vi "test_LoadFrameEditorFile_v2.vi"(11 "BIN file path":path=path "C:/Users/Administrator/Desktop/git/niveristand-aim-arinc664-custom-device/Docs/User Guide/Assets/standard_frames_udp.bin") -> (0 "error out":errorcluster)   [LabVIEW 2020]
uses:
  <instrlib>/AIM GmbH/_AIM 664/helpers/EthFrameManagement/EthFrameManagement.lvlib
  Frame Configuration/controls/Type of Payload.ctl
  Frame Configuration/controls/Payload Record Type.ctl
  Import/AIM ARINC 664 Import.lvlib
  <instrlib>/AIM GmbH/_AIM 664/helpers/EthFrameManagement/controls/ehternetFrame_type.ctl
  <instrlib>/AIM GmbH/_AIM 664/helpers/EthFrameManagement/controls/IPFrame_type.ctl
  <instrlib>/AIM GmbH/_AIM 664/helpers/EthFrameManagement/controls/UDPFrame_type.ctl
  Shared/frame_tx_generic_seqNumberInit.ctl
  Shared/frame_tx_generic_seqNumberOffset.ctl
  Shared/frame_tx_generic.ctl
  <vilib>/NI/NI VeriStand Encoding and Decoding/Encoding.ctl
  <vilib>/NI/NI VeriStand Encoding and Decoding/Encoding and Decoding.lvlib
  Shared/frame_parameter_definition.ctl
  Shared/frame_parameter.ctl
panel:
  out "Frame Headers":T1[](array[typedef]) {"Frame header"."SequenceNumberOffset" items=["FDX_TX_FRAME_SEQ_OFFS_AUTO"=65535]; "Frame header"."SequenceNumberInit" items=["FDX_TX_FRAME_SEQ_INIT_AUTO"=65535, "FDX_TX_FRAME_SEQ_OFF"=65533]; "Frame header"."PhysErrorInjection" items=["FDX_TX_FRAME_ERR_OFF", "FDX_TX_FRAME_ERR_CRC", "FDX_TX_FRAME_ERR_ALI", "FDX_TX_FRAME_ERR_PRE", "FDX_TX_FRAME_ERR_PHY"]; "Frame header"."PayloadGenerationMode" items=["FDX_TX_FRAME_PGM_USER", "FDX_TX_FRAME_PGM_IP_PART", "FDX_TX_FRAME_PGM_IP_PART_TT", "FDX_TX_FRAME_PGM_IP_FULL", "FDX_TX_FRAME_PGM_IP_FULL_TT"]; "Frame header"."PayloadBufferMode" items=["FDX_TX_FRAME_PBM_STD", "FDX_TX_FRAME_PBM_MAC", "FDX_TX_FRAME_PBM_UDP", "FDX_TX_FRAME_PBM_FULL"]; "Frame header"."NetSelect" items=["FDX_TX_FRAME_DLY_A"=0, "FDX_TX_FRAME_DLY_B"=1, "FDX_TX_FRAME_BOTH "=3, "FDX_TX_FRAME_ONLY_A"=4, "FDX_TX_FRAME_ONLY_B "=5]; "Frame header"."FrameStartMode" items=["FDX_TX_FRAME_START_IFG", "FDX_TX_FRAME_START_PGWT", "FDX_TX_FRAME_START_TRG", "FDX_TX_FRAME_START_TRG_D"]}
  in  "port index":i32
  in  "frame index":i32
  in  "XML file path":path=path "C:/Users/Administrator/Desktop/git/niveristand-aim-arinc664-custom-device/Docs/User Guide/Assets/Loopback_TxGen_RxMonitor.xml"
  out "data":cluster{"FrameID":string, "frame_record":T7}[](array[cluster])=[{"FrameID"="Payload1", "frame_record"={"Data"=[3, 0, 0, 0, 0, 60, 2, 0, 0, 1, 33, 32, 8, 0, 69, 0, 0, 45, 0, 0, 64, 0, 1, 17, 109, 162, 10, 1, 33, 1, 224, 224, 0, 60, 0, 1, 0, 1, 0, 25, 0, 0, 0, 0, 0, 0, 0, 0, 0, 0, 0, 0, 0, 0, 0, 0, 0, 0, 0, 0, 0, 0, 0, 0], "Type of Frame"=1}}, {"FrameID"="Payload2", "frame_record"={"Data"=[3, 0, 0, 0, 0, 60, 2, 0, 0, 1, 33, 32, 8, 0, 69, 0, 0, 45, 0, 0, 64, 0, 1, 17, 109, 162, 10, 1, 33, 1, 224, 224, 0, 60, 0, 1, 0, 1, 0, 25, 0, 0, 65, 66, 67, 68, 69, 70, 71, 72, 73, 74, 75, 76, 77, 78, 79, 80, 81, 0, 0, 0, 0, 0], "Type of Frame"=1}}, {"FrameID"="Payload3", "frame_record"={"Data"=[10, 10, 10, 10, 10, 10, 10, 10, 10, 10, 10, 10, 10, 10, 10, 10, 10], "Type of Frame"=2}}] {"frame_record"."Type of Frame" items=["Raw Frame", "UDP/IP Tx Gen", "Tx UDP"]; "frame_record"."Data" format="%.0x"}
  out "dst ip":string="224.224.0.60"
  out "src ip":string="10.1.33.1"
  out "size(s)":i32=22
  out "UDP header":T9={"Source Port"=1, "Dest Port"=1, "Lenght"=25, "Checksum"=0}
  out "IP header":T10={"Version"=4, "IHL"=5, "ToS"=0, "Length"=45, "ID"=0, "CtlFlags"=2, "FragOffset"=0, "TTL"=1, "Protocol"=17, "Checksum"=28066, "Source IP"=167846145, "Dest IP"=3772776508} {"CtlFlags" format="%.0b"; "Dest IP" format="%.0x"; "Source IP" format="%.0x"; "Checksum" format="%.0x"; "TTL" format="%.0x"; "FragOffset" format="%.0x"; "ID" format="%.0x"; "Length" format="%.0x"; "ToS" format="%.0x"; "IHL" format="%.0x"; "Version" format="%.0x"}
  out "UDP Header Only":u8[](array[numeric])=[0, 1, 0, 1, 0, 25, 0, 0]
  out "IP Header Only":u8[](array[numeric])=[69, 0, 0, 45, 0, 0, 64, 0, 1, 17, 109, 162, 10, 1, 33, 1, 224, 224, 0, 60] format="%.0x"
  out "Ethernet header":T11={"Dest MAC"=[3, 0, 0, 0, 0, 60], "Src MAC"=[2, 0, 0, 1, 33, 32], "EtherType"=2048} {"EtherType" format="%04x"; "Src MAC" format="%02x"; "Dest MAC" format="%.0b"}
  out "MAC Header Only":u8[](array[numeric])=[3, 0, 0, 0, 0, 60, 2, 0, 0, 1, 33, 32, 8, 0] format="%.0x"
  out "payload":u8[](array[numeric]) format="%.0x"
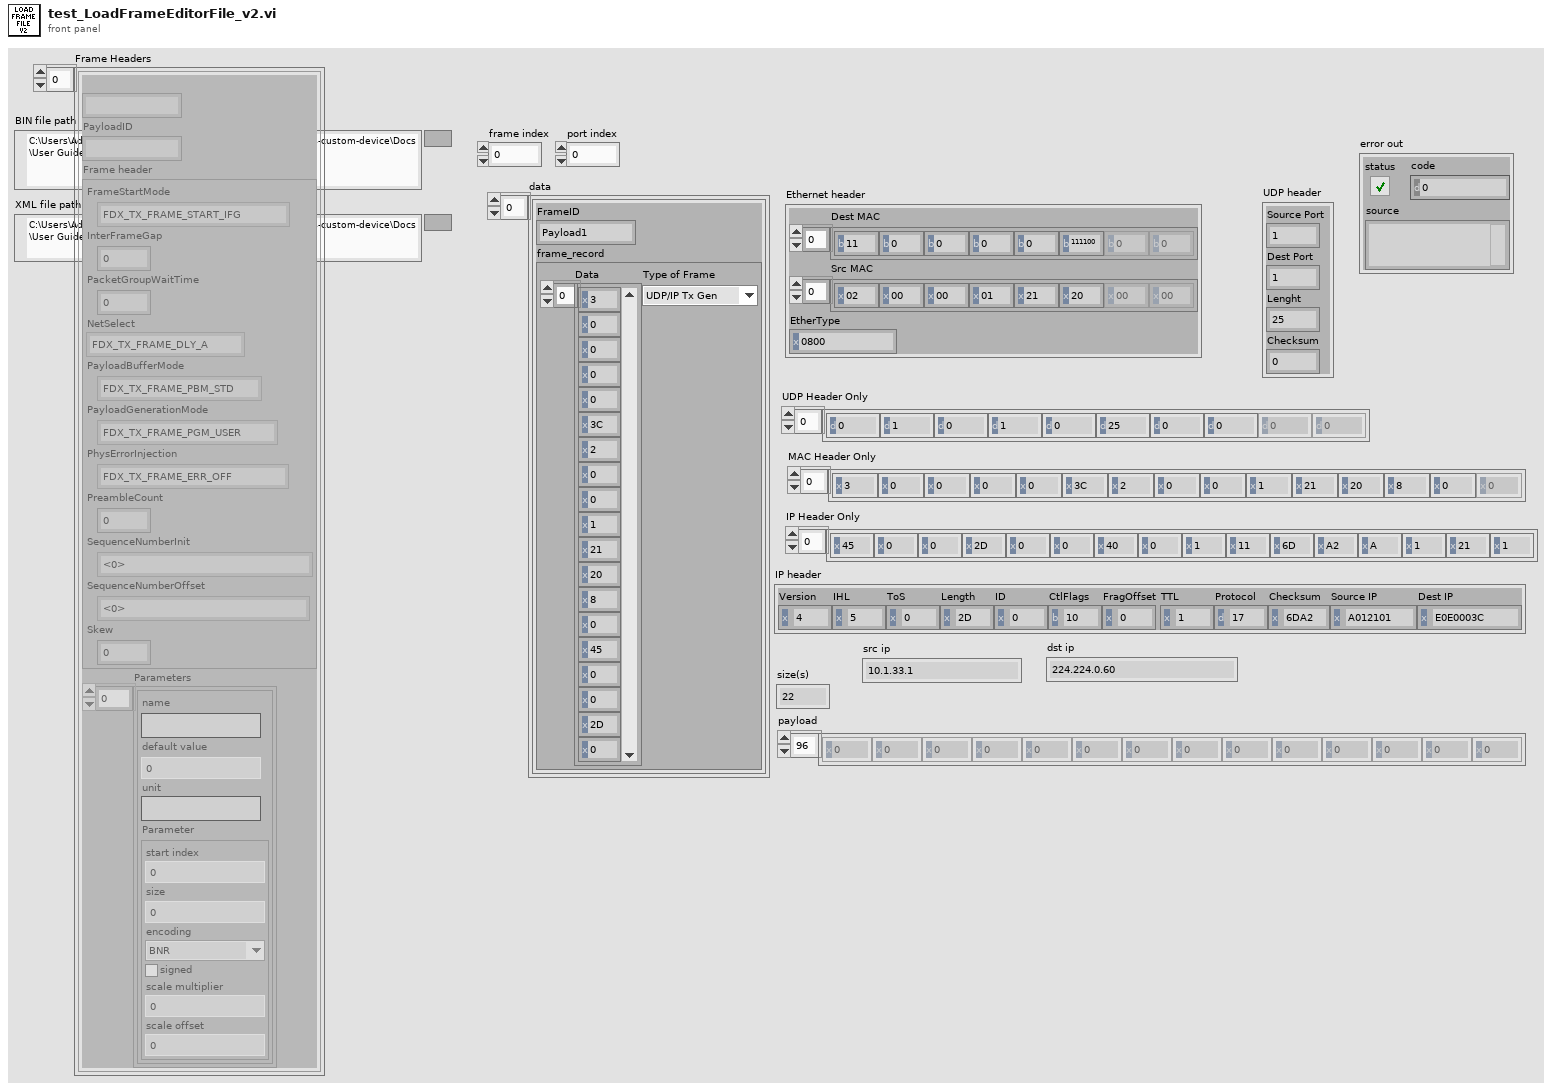
[diagram p1: front panel]
types:
  T1 = typedef "AIM ARINC 664 Import.lvlib/frame_tx_generic.ctl" = cluster{"FrameID":string, "PayloadID":string, "Frame header":cluster{"FrameStartMode":i32, "InterFrameGap":i32, "PacketGroupWaitTime":i32, "NetSelect":u32, "PayloadBufferMode":i32, "PayloadGenerationMode":i32, "PhysErrorInjection":i32, "PreambleCount":i32, "SequenceNumberInit":T2, "SequenceNumberOffset":T3, "Skew":i32}, "Parameters":T4[]}
  T2 = typedef "AIM ARINC 664 Import.lvlib/frame_tx_generic_seqNumberInit.ctl" = i32
  T3 = typedef "AIM ARINC 664 Import.lvlib/frame_tx_generic_seqNumberOffset.ctl" = i32
  T4 = typedef "AIM ARINC 664 Import.lvlib/frame_parameter.ctl" = cluster{"name":string, "default value":dbl, "unit":string, "Parameter":T5}
  T5 = typedef "AIM ARINC 664 Import.lvlib/frame_parameter_definition.ctl" = cluster{"start index":i32, "size":i32, "encoding":T6, "signed":bool, "scale multiplier":dbl, "scale offset":dbl}
  T6 = typedef "Encoding and Decoding.lvlib/Encoding.ctl" = enum16{"BNR", "BCD", "Discrete"}
  T7 = typedef "Payload Record Type.ctl" = cluster{"Data":u8[], "Type of Frame":T8}
  T8 = typedef "Type of Payload.ctl" = u16
  T9 = typedef "EthFrameManagement.lvlib/UDPFrame_type.ctl" = cluster{"Source Port":u16, "Dest Port":u16, "Lenght":u16, "Checksum":u16}
  T10 = typedef "EthFrameManagement.lvlib/IPFrame_type.ctl" = cluster{"Version":u8, "IHL":u8, "ToS":u8, "Length":u16, "ID":u16, "CtlFlags":u8, "FragOffset":u16, "TTL":u8, "Protocol":u8, "Checksum":u16, "Source IP":u32, "Dest IP":u32}
  T11 = typedef "EthFrameManagement.lvlib/ehternetFrame_type.ctl" = cluster{"Dest MAC":u8[], "Src MAC":u8[], "EtherType":u16}
  T12 = typedef "AIM ARINC 664 Import.lvlib/Board Top Level Configuration.ctl" = cluster{"boardSetup":T13, "portConfiguration":T14[]}
  T13 = typedef "AIM ARINC 664 Import.lvlib/board_setup.ctl" = cluster{"boardId":u32, "portSpeed":u32, "portConfig":u32}
  T14 = typedef "AIM ARINC 664 Import.lvlib/port_configuration.ctl" = cluster{"portSetup":T15, "Tx_Generic":T16[], "Rx_Monitor":cluster{"DefaultCronoMode":u32, "GlbMonBufferSizeIn":u32, "CaptureMode":u32, "MaxFileSizeMB":u32, "Strobe":u32, "TriggerPosition":u32}[], "Tx_UDP":cluster{"tx_udp_setup":cluster{"VlId":i32, "Bag":i32, "NetSelect":u32, "domainID":u8, "sideID":u8, "locationID":u8, "interfaceID":u8, "NumOfSubVl":u16, "Skew":u32, "MaxFrameLength":u32, "FrameBufferSize":u32}, "commPorts":T18[], "sapPorts":T19[]}[], "Rx_UDP":cluster{"Tx_UDP":T20, "commPorts":T21[], "sapPorts":T22[]}[]}
  T15 = typedef "AIM ARINC 664 Import.lvlib/port_setup.ctl" = cluster{"port Id":u32, "redundant":bool}
  T16 = typedef "AIM ARINC 664 Import.lvlib/session_tx_generic.ctl" = cluster{"tx_generic_setup":T17, "Frame Headers":T1[]}
  T17 = typedef "AIM ARINC 664 Import.lvlib/tx_generic_setup.ctl" = cluster{"QueueSizeIn":u32, "Count":i32, "StartMode":i32}
  T18 = typedef "AIM ARINC 664 Import.lvlib/port_tx_udp_comm.ctl" = cluster{"PayloadID":string, "partitionID":u8, "UdpSrcPort":u16, "UdpDstPort":u16, "PortType":enum16{"FDX_UDP_SAMPLING", "FDX_UDP_QUEUING"}, "SubVIId":u32, "UdpNumBufMessages":u32, "UdpMaxMessageSize":u32, "UdpSamplingRate":u32, "Parameters":T4[]}
  T19 = typedef "AIM ARINC 664 Import.lvlib/port_tx_udp_sap.ctl" = cluster{"PayloadID":string, "SubVlId":u8, "UdpSrcPort":u16, "UdpNumBufMessages":u32, "UdpMaxMessageSize":u32, "partitionID":u8, "domainID":u8, "sideID":u8, "locationID":u8, "interfaceID":u8, "Parameters":T4[]}
  T20 = typedef "AIM ARINC 664 Import.lvlib/rx_udp_setup.ctl" = cluster{"VerificationMode":u32, "Bag":u32, "Jitter":u32, "MaxFrameLength":u32, "MaxSkew":u32, "VLBufSize":u32, "FilterMode":u32, "FilterPosition":u32, "Padding":u32, "FilterMask":u32, "FilterData":u32, "MinFrameLength":u32, "VlId":u16, "VLRange":u32}
  T21 = typedef "AIM ARINC 664 Import.lvlib/port_rx_udp_comm.ctl" = cluster{"PayloadID":string, "domainID":u8, "sideID":u8, "locationID":u8, "partitionID":u8, "UdpSrcPort":u16, "UdpDstPort":u16, "PortType":enum16{"FDX_UDP_SAMPLING", "FDX_UDP_QUEUING"}, "SubVIId":u32, "UdpNumBufMessages":u32, "UdpMaxMessageSize":u32, "UdpSamplingRate":u32, "Parameters":T4[]}
  T22 = typedef "AIM ARINC 664 Import.lvlib/port_rx_udp_sap.ctl" = cluster{"PayloadID":string, "UdpDstPort":u16, "UdpNumBufMessages":u32, "UdpMaxMessageSize":u32, "Parameters":T4[]}
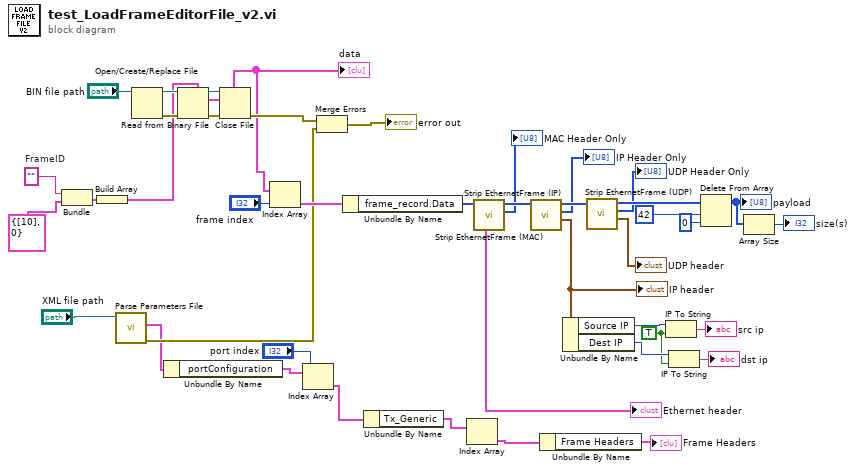
[diagram p0: block diagram]
diagram:
  w14 = ""  # FrameID
  w18 = TRUE ("dot notation? (F)")
  n1 = Bundle("FrameID"=w14, "frame_record"=T7 {"Data"=[10], "Type of Frame"=0}) -> (w13:cluster{"FrameID":string, "frame_record":T7})  [unwired: 1 in]
  n2 = Build Array(w13) -> (w12:cluster{"FrameID":string, "frame_record":T7}[])
  n3 = call "Parse Parameters File.vi"("path to XML document"="XML file path") -> ("error out"=w9:errorcluster, "board configuration out"=w8:T12)  [unwired: 8 in, 1 out]
  n4 = Open/Create/Replace File(file path (use dialog)="BIN file path") -> (refnum out=w40:refnum<file>, error out=w39:errorcluster)  [unwired: 5 in, 1 out]
  n5 = Unbundle By Name(w8) -> ("portConfiguration"=w7:T14[])
  n6 = Read from Binary File(5:w12, 8:w39, 11:w40) -> (0:w41:errorcluster, 2:w36:cluster{"FrameID":string, "frame_record":T7}[], 3:w42:refnum<file>)  [unwired: 3 in, 1 out]
  "data" <- w36
  n7 = Close File(refnum=w42, error in=w41) -> (error out=w38:errorcluster)  [unwired: 1 out]
  n8 = Index Array(array=w36, index="frame index") -> (element=w35:cluster{"FrameID":string, "frame_record":T7})
  n9 = Index Array(array=w7, index="port index") -> (element=w5:T14)
  n10 = Merge Errors(w38, w9) -> (→"error out":errorcluster)
  n11 = Unbundle By Name(w35) -> ("frame_record.Data"=w34:u8[])
  n12 = Unbundle By Name(w5) -> ("Tx_Generic"=w3:T16[])
  n13 = Index Array(array=w3) -> (element=w2:T16)  [unwired: 1 in]
  n14 = call <instrlib>:"Strip EthernetFrame (MAC).vi"("Ethernet Frame In"=w34) -> ("Ethernet header"=→"Ethernet header":T11, "MAC Header Only"=→"MAC Header Only":u8[], "Ethernet Frame Out"=w33:u8[])  [unwired: 7 in, 1 out]
  n15 = call <instrlib>:"Strip EthernetFrame (IP).vi"("Frame In"=w33) -> ("IP header"=w21:T10, "IP Header Only"=→"IP Header Only":u8[], "Frame Out"=w32:u8[])  [unwired: 7 in, 1 out]
  "IP header" <- w21
  n16 = Unbundle By Name(w2) -> ("Frame Headers"=→"Frame Headers":T1[])
  n17 = Unbundle By Name(w21) -> ("Source IP"=w20:u32, "Dest IP"=w19:u32)
  n18 = call <instrlib>:"Strip EthernetFrame (UDP).vi"("Ethernet Frame In"=w32) -> ("UDP header"=→"UDP header":T9, "UDP Header Only"=→"UDP Header Only":u8[], "Ethernet Frame Out"=w31:u8[])  [unwired: 7 in, 1 out]
  n19 = IP To String(1:w18, 2:w20) -> (0:→"src ip":string)
  n20 = IP To String(1:w18, 2:w19) -> (0:→"dst ip":string)
  n21 = Delete From Array(array=w31, length=42 ("index"), index=0) -> (array with subset deleted=w23:u8[])  [unwired: 1 out]
  "payload" <- w23
  n22 = Array Size(array=w23) -> (size(s)=→"size(s)":i32)
